vi "GetText.vi"(8 "error in":errorcluster, 11 "group in":refnum<class "device.lvclass">) -> (0 "error out":errorcluster, 1 "additional text":string, 2 "text":string, 3 "group out":refnum<class "device.lvclass">, 4 "glyph":string)   [LabVIEW 2013, in "device.lvclass"]
uses:
  device.lvclass
  device.lvclass/device.ctl
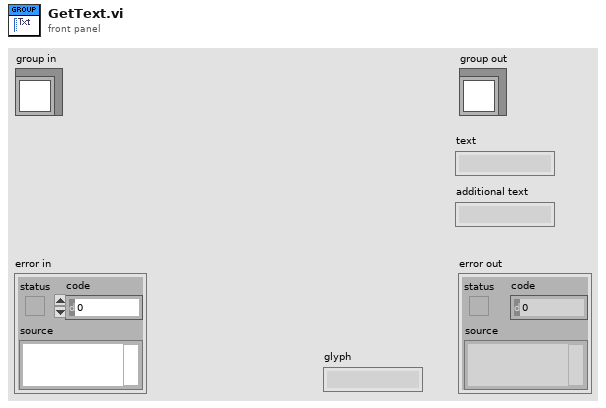
[diagram p1: front panel]
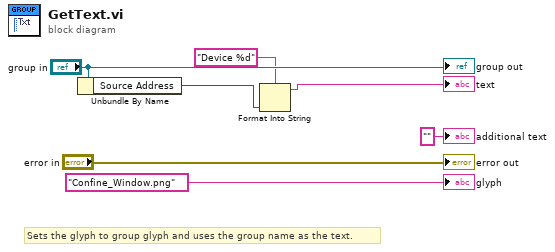
[diagram p0: block diagram]
diagram:
  # "Sets the glyph to group glyph and uses the group name as the text."
  n1 = Unbundle By Name("group in") -> ("Source Address"=w3:u8)
  n2 = Format Into String(format string="Device %d", w3) -> (resulting string=→"text":string)  [unwired: 2 in, 1 out]
  "error out" <- "error in"
  "group out" <- "group in"
  "additional text" <- "" ("additional text")
  "glyph" <- "Confine_Window.png" ("glyph")
